vi "ADD ITEM TO PGSQL.vi"(9 "ITEM DATA IN":T1) -> (1 "ITEM DATA OUT":T1)   [LabVIEW 2019]
uses:
  Controls/Table Data Types/Inventory Data Type.ctl
  <vilib>/addons/database/Connection.llb/DB Tools Open Connec (String).vi
  <vilib>/addons/database/NI_Database_API.lvlib
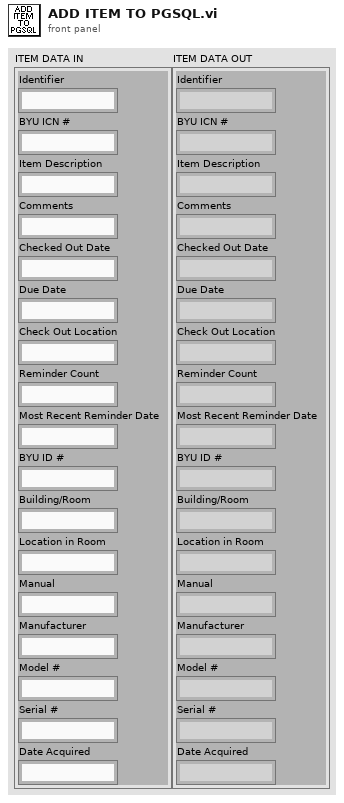
[diagram p1: front panel]
types:
  T1 = cluster{"Identifier":string, "BYU ICN #":string, "Item Description":string, "Comments":string, "Checked Out Date":string, "Due Date":string, "Check Out Location":string, "Reminder Count":string, "Most Recent Reminder Date":string, "BYU ID #":string, "Building/Room":string, "Location in Room":string, "Manual":string, "Manufacturer":string, "Model #":string, "Serial #":string, "Date Acquired":string}
  T2 = typedef "Inventory Data Type.ctl" = cluster{"Identifier":string, "BYU ICN #":string, "Item Description":string, "Comments":string, "Checked Out Date":string, "Due Date":string, "Check Out Location":string, "Reminder Count":i32, "Most Recent Reminder Date":string, "BYU ID #":string, "Building/Room":string, "Location in Room":string, "Manual":string, "Manufacturer":string, "Model #":string, "Serial #":string, "Date Acquired":string}
  T3 = typedef "NI_Database_API.lvlib/Conn ObjectReference.ctl" = refnum<k1>
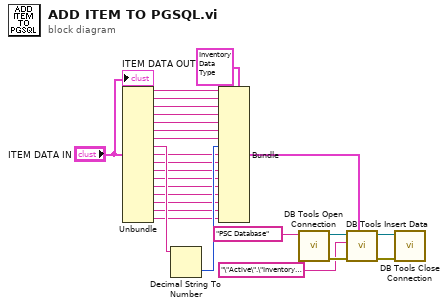
[diagram p0: block diagram]
diagram:
  n1 = Unbundle("ITEM DATA IN") -> ("Identifier"=w26:string, "BYU ICN #"=w25:string, "Item Description"=w24:string, "Comments"=w23:string, "Checked Out Date"=w22:string, "Due Date"=w21:string, "Check Out Location"=w20:string, "Reminder Count"=w19:string, "Most Recent Reminder Date"=w17:string, "BYU ID #"=w16:string, "Building/Room"=w15:string, "Location in Room"=w14:string, "Manual"=w13:string, "Manufacturer"=w12:string, "Model #"=w11:string, "Serial #"=w10:string, "Date Acquired"=w9:string)
  n2 = Decimal String To Number(string=w19) -> (number=w18:i32)  [unwired: 2 in, 1 out]
  n3 = Bundle(cluster=T2 {"Identifier"="", "BYU ICN #"="", "Item Description"="", "Comments"="", "Checked Out Date"="", "Due Date"="", "Check Out Location"="", "Reminder Count"=0, "Most Recent Reminder Date"="", "BYU ID #"="", "Building/Room"="", "Location in Room"="", "Manual"="", "Manufacturer"="", "Model #"="", "Serial #"="", "Date Acquired"=""} ("INVENTORY DATA TYPE"), "Identifier"=w26, "BYU ICN #"=w25, "Item Description"=w24, "Comments"=w23, "Checked Out Date"=w22, "Due Date"=w21, "Check Out Location"=w20, "Reminder Count"=w18, "Most Recent Reminder Date"=w17, "BYU ID #"=w16, "Building/Room"=w15, "Location in Room"=w14, "Manual"=w13, "Manufacturer"=w12, "Model #"=w11, "Serial #"=w10, "Date Acquired"=w9) -> (w3:T2)
  n4 = call-poly <vilib>:"DB Tools Open Connection.vi"("connection information"="PSC Database") -> ("error out"=w5:errorcluster, "connection reference"=w6:T3)  [unwired: 7 in]
  n5 = call <vilib>:"DB Tools Insert Data.vi"("data"=w3, "error in (no error)"=w5, "table"="\"Active\".\"Inventory\"", "connection reference"=w6) -> ("error out"=w2:errorcluster, "connection reference out"=w1:T3)  [unwired: 6 in]
  n6 = call <vilib>:"DB Tools Close Connection.vi"("error in (no error)"=w2, "connection reference"=w1) -> ()  [unwired: 5 in, 1 out]
  "ITEM DATA OUT" <- "ITEM DATA IN"
